vi "Test Power Supply API.vi"() -> ()   [LabVIEW 2025, in "Power Supply.lvlib"]
doc: "Power Supply API Tester.\n\n<b>Note:</b> This VI was modified by the <b>Validate DQMH Module</b> tool to add the 'Show Main VI Diagram on Init' functionality included in DQMH 6.1.\n\n<b>Note:</b> This VI was modified by the <b>Validate DQMH Module</b> tool to upgrade it to the DQMH 5.0 approach to only call the Stop Module.vi at the end of the tester if the module wasn't originally running when the tester started.\n\n<b>Note:</b> This VI was modified by the <b>Validate DQMH Module</b> tool to remove code to stop the main loop on error, and instead display the most recent error on the tester front panel.\n\n<b>Note:</b> This VI was modified by the <b>Validate DQMH Module</b> tool to upgrade its Error Reported event frame to use an improved mechanism for displaying error information."
uses:
  Power Supply.lvlib
  <vilib>/MGI/Panel Manager/Panel/Panel.lvlib
  <vilib>/MGI/Panel Manager/Panel/Panel/Window/Window.vi
  <vilib>/MGI/Panel Manager/Panel/Panel/Window/Window.lvclass
  <vilib>/MGI/Panel Manager/Panel/Panel/Subpanel/Subpanel.vi
  <vilib>/MGI/Panel Manager/Panel/Panel/Subpanel/Subpanel.lvclass
  <vilib>/MGI/Panel Manager/Panel/Panel/Window/Dialog/Dialog.vi
  <vilib>/MGI/Panel Manager/Panel/Panel/Window/Dialog/Dialog.lvclass
  <vilib>/Utility/error.llb/DialogType.ctl
  DC Output--enum.ctl
  Function Generator State--cluster.ctl
  Function Generator Parameters--cluster.ctl
panel:
  in  "Function Generator":T1
  in  "Set Function Generator Parameters":bool
  in  "Function Generator State":T2
  in  "Set Function Generator State":bool
  in  "Disconnect":bool
  in  "Connect":bool
  out "last error":errorcluster
  in  "Show Main VI Diagram on Init (F)":bool
  out "Power Supply State":map{string, dbl}(c390)
  in  "DC Ouput":T3
  in  "Set DC Output":bool
  in  "Plugin File Path":path
  in  "Set Power Supply Plugin":bool
  in  "Power [W]":dbl
  in  "Set Power SP":bool
  in  "Voltage SP [V]":dbl
  in  "Set Voltage SP":bool
  in  "Current SP [A]":dbl
  in  "Set Current SP":bool
  in  "Autoshow?":bool
  in  "Panel Type":enum16{"Window", "Dialog", "Subpanel"}(ring)
  in  "Change Panel":bool
  in  "Tab Control":enum32{"Status", "Subpanel"}(tab)
  out "Status":string
  in  "Show Block Diagram":bool
  in  "Stop Module":bool
  in  "Start Module":bool
  in  "Hide Module Panel":bool
  in  "Show Module Panel":bool
  out "Module Running?":bool
  # "This VI tests the API for the Module."
  # "Change Panel"
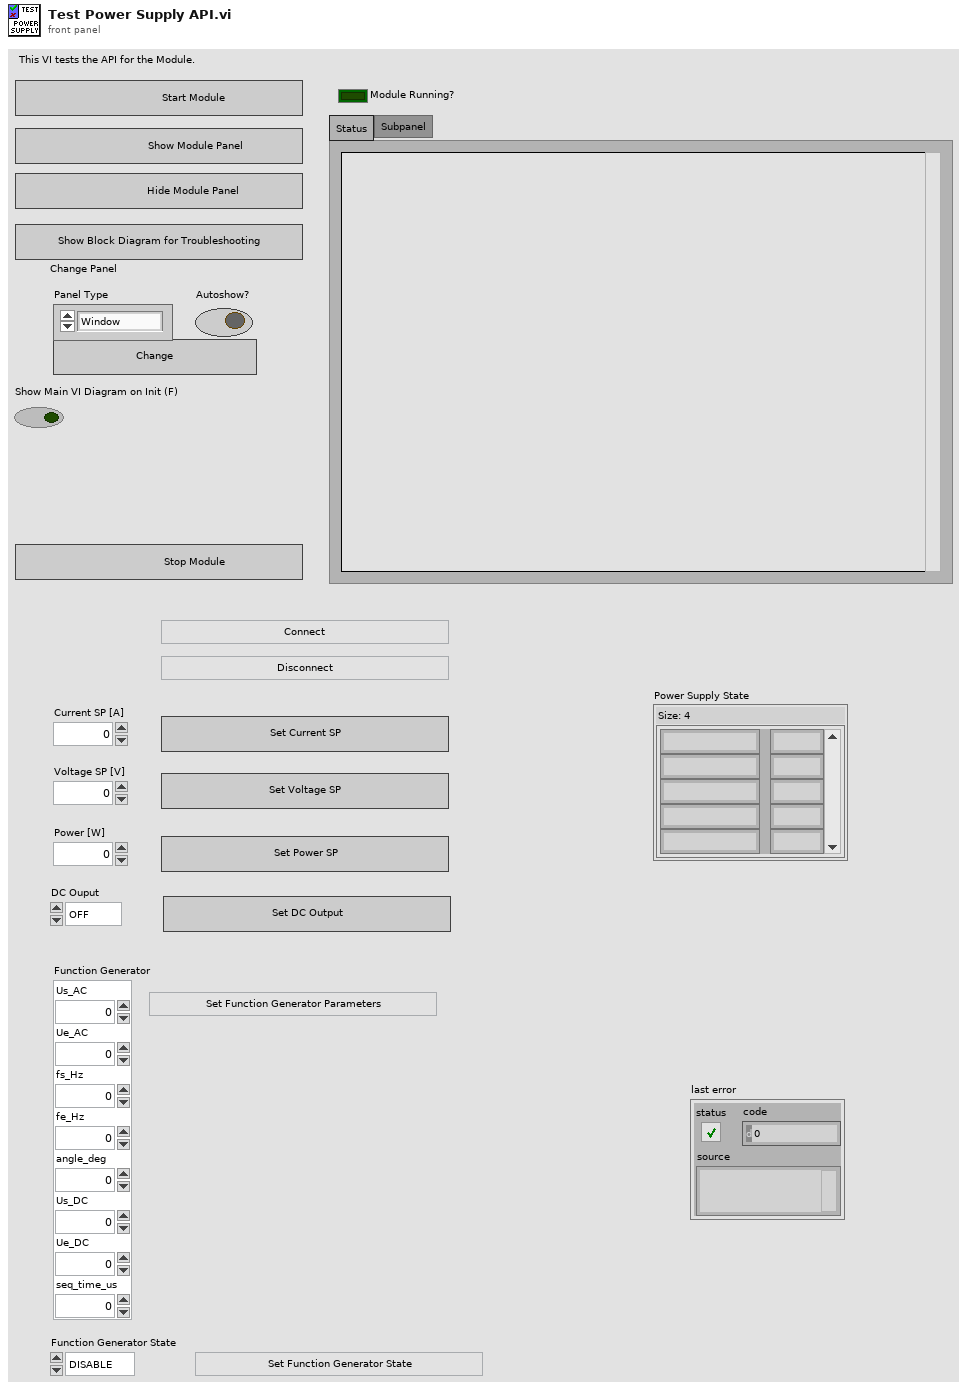
[diagram p1: front panel]
types:
  T1 = typedef "Power Supply.lvlib/Function Generator Parameters--cluster.ctl" = cluster{"Us_AC":sgl, "Ue_AC":sgl, "fs_Hz":sgl, "fe_Hz ":sgl, "angle_deg ":sgl, "Us_DC ":sgl, "Ue_DC":sgl, "seq_time_us":sgl}
  T2 = typedef "Power Supply.lvlib/Function Generator State--cluster.ctl" = enum16{"DISABLE", "ENABLE"}
  T3 = typedef "Power Supply.lvlib/DC Output--enum.ctl" = enum16{"OFF", "ON"}
  T4 = typedef "Power Supply.lvlib/Broadcast Events--cluster.ctl" = cluster{"Module Did Init":refnum<user-event>, "Status Updated":refnum<user-event>, "Error Reported":refnum<user-event>, "Module Did Stop":refnum<user-event>, "Update Module Execution Status":refnum<user-event>, "Broadcast Power Supply State":refnum<user-event>}
  T5 = typedef "DialogType.ctl" = u16
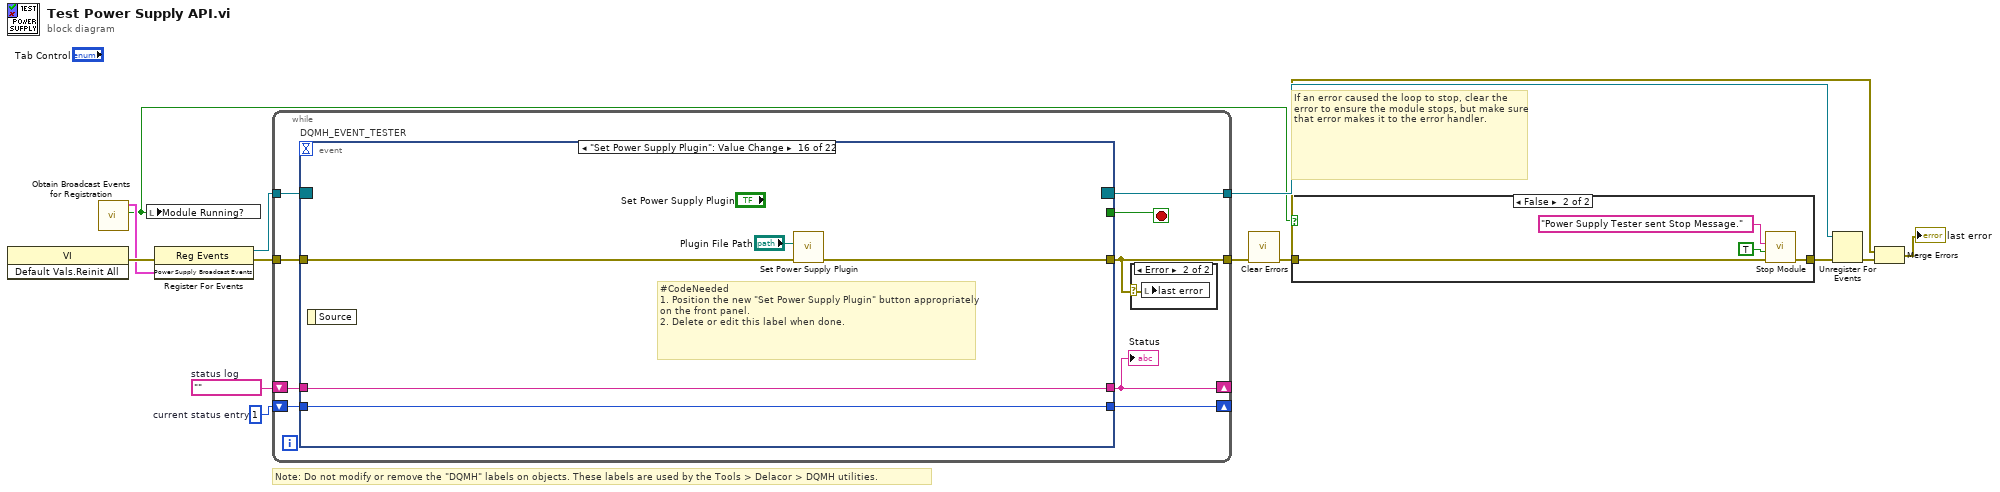
[diagram p0: block diagram]
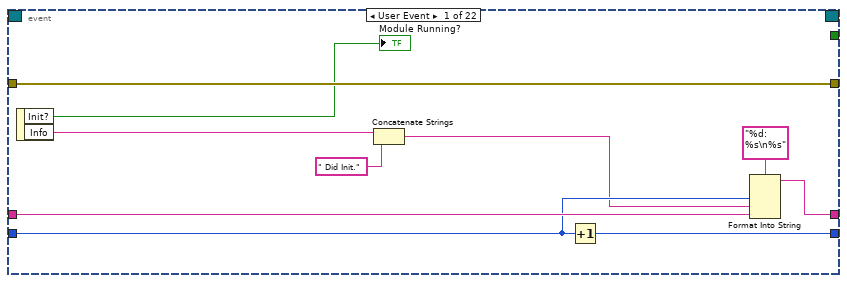
[diagram p4: hidden frame]
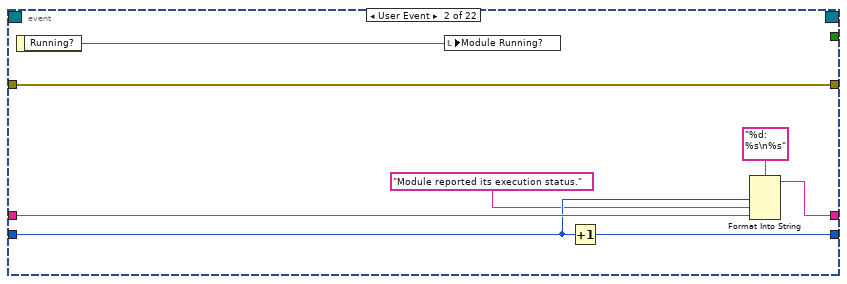
[diagram p5: hidden frame]
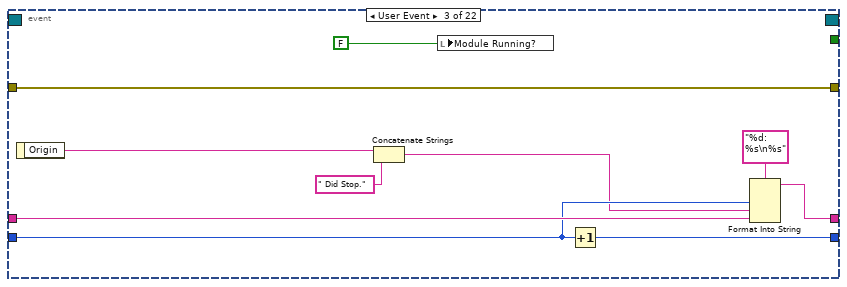
[diagram p6: hidden frame]
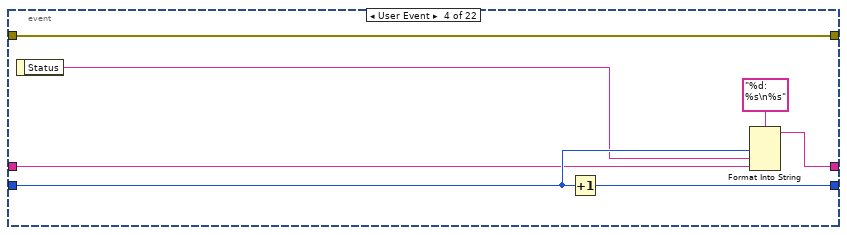
[diagram p7: hidden frame]
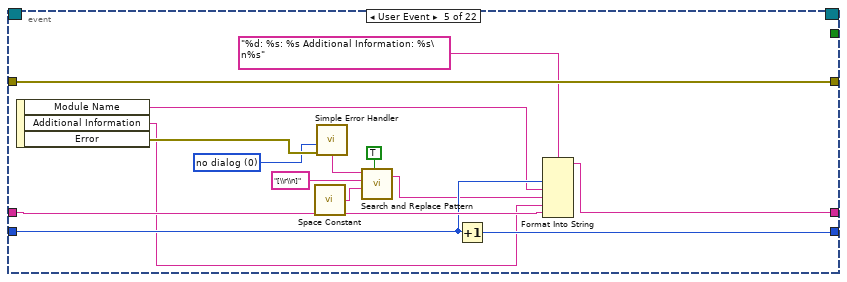
[diagram p8: hidden frame]
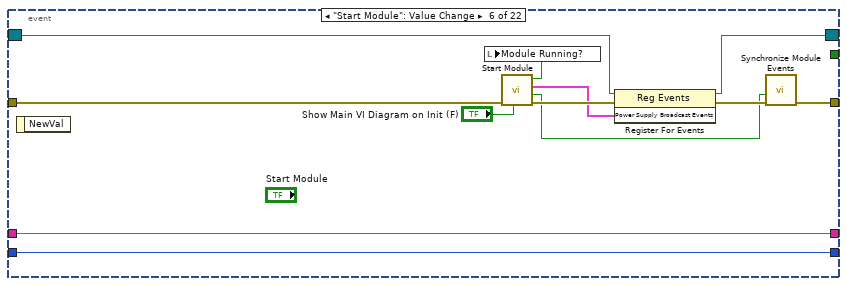
[diagram p9: hidden frame]
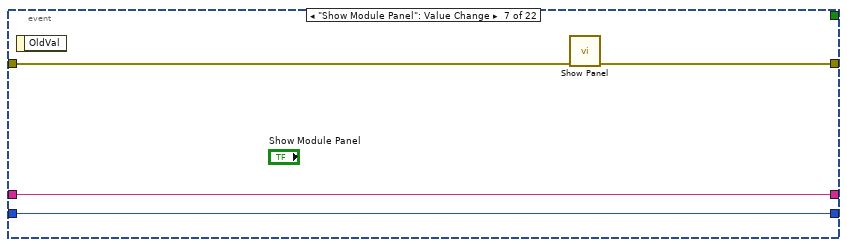
[diagram p10: hidden frame]
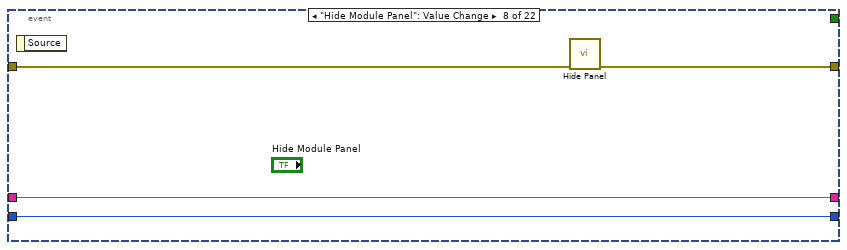
[diagram p11: hidden frame]
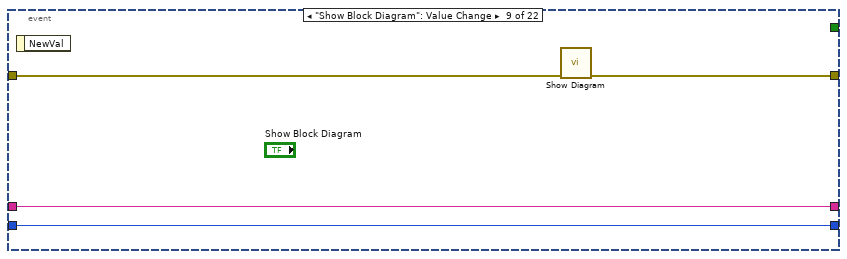
[diagram p12: hidden frame]
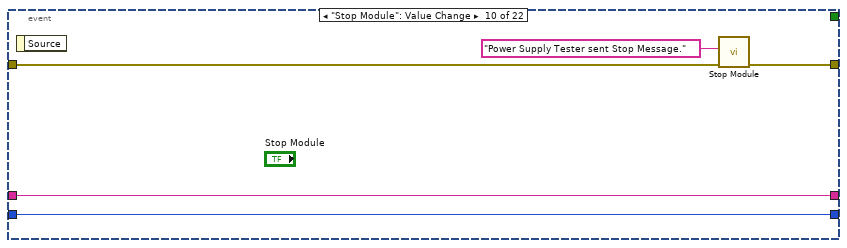
[diagram p13: hidden frame]
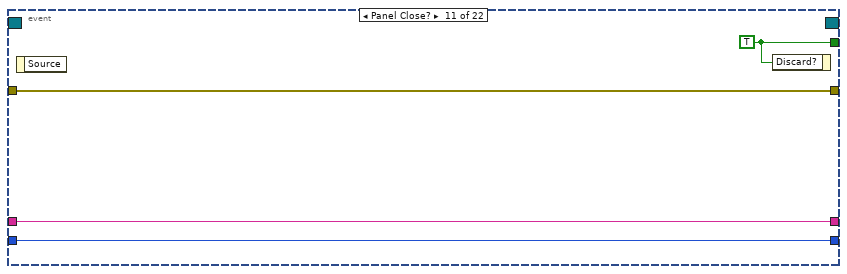
[diagram p14: hidden frame]
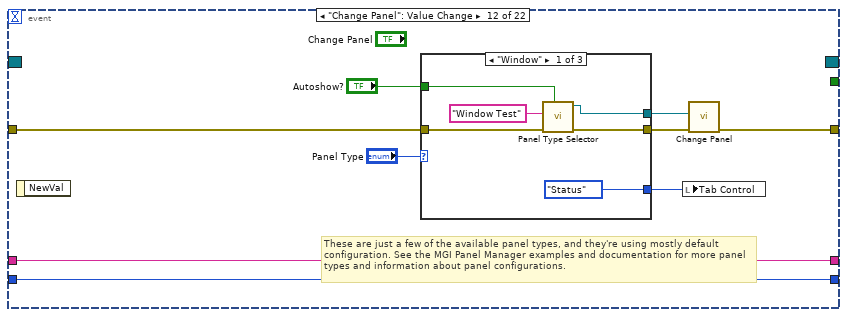
[diagram p15: hidden frame]
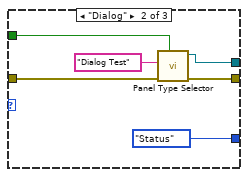
[diagram p16: hidden frame]
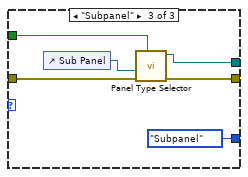
[diagram p17: hidden frame]
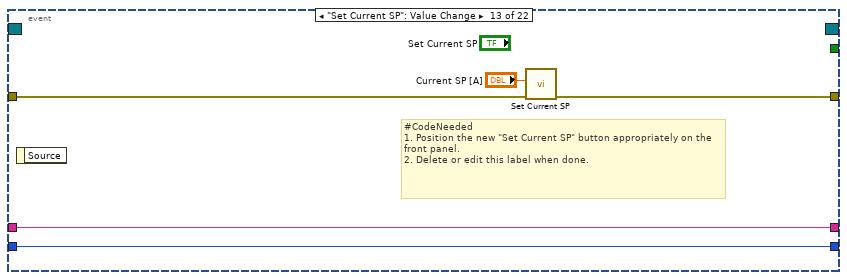
[diagram p18: hidden frame]
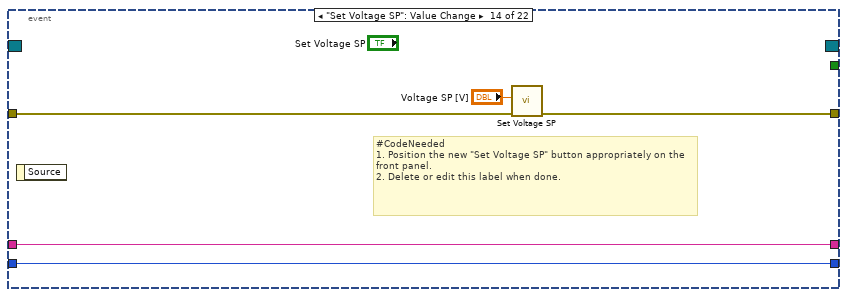
[diagram p19: hidden frame]
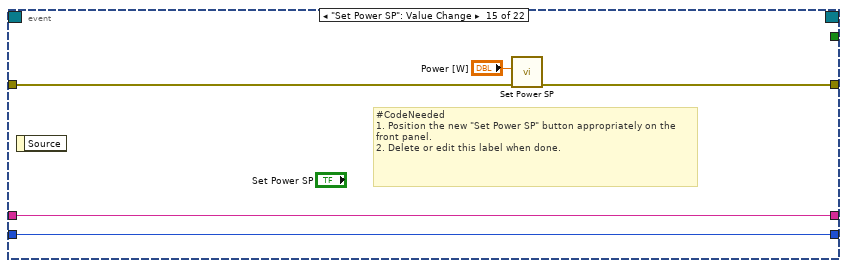
[diagram p20: hidden frame]
diagram:
  w10 = 1  # current status entry
  w11 = ""  # status log
  # "If an error caused the loop to stop, clear the error to ensure the module stops, but make sure that error makes it to the error handler."
  # "Note: Do not modify or remove the \"DQMH\" labels on objects. These labels are used by the Tools > Delacor > DQMH utilities."
  n1 = invoke class="VI" method="Default Vals.Reinit All"() -> (error out=w9:errorcluster)  [unwired: 3 in, 2 out]
  n2 = call "Obtain Broadcast Events for Registration.vi"() -> ("Already running?"=w2:bool, "Power Supply Broadcast Events"=w7:T4)  [unwired: 9 in, 1 out]
  n3 = local write "Module Running?"(w2) -> ()
  n4 = register-events(error in=w9, w7) -> (reference out=w6:refnum<event-registration>, error out=w8:errorcluster)  [unwired: 1 in]
  n5 = while {
    tunnel: w6 -> [w22]
    tunnel: [w15] -> w3
    shift-right: [w18] -> _
    shift-left: w11 -> [w20]
    shift-right: [w19] -> _
    shift-left: w10 -> [w21]
    tunnel: w8 -> [w17]
    tunnel: [w16] -> w5
    stop <- w14 stop-if-true
    n6 = event "DQMH_EVENT_TESTER" shown="[15] \"Set Power Supply Plugin\": Value Change" {
      selector: w22 -> [_ _ _ _ _ w79 _ _ _ _ _ _ _ _ _ _ _ _ _ _ _ _]
      dyn-events: [_ _ _ _ _ w78 _ _ _ _ _ _ _ _ _ _ _ _ _ _ _ _] -> w16
      timeout: _ -> [_ _ _ _ _ _ _ _ _ _ _ _ _ _ _ _ _ _ _ _ _ _]
      tunnel: [_ _ _ _ _ _ _ _ _ _ w106 _ _ _ _ _ _ _ _ _ _ _] -> w14
      tunnel: [w33 w35 w42 w52 w73 w77 w89 w93 w94 w100 w103 w113 w135 w140 w145 w150 w155 w168 w169 w173 w178 w183] -> w15
      tunnel: w21 -> [w29 w39 w49 w55 w70 w82 w87 w91 w95 w101 w104 w114 w136 w141 w146 w151 w156 w165 w170 w174 w179 w184]
      tunnel: w20 -> [w30 w40 w50 w54 w72 w83 w88 w92 w96 w102 w105 w115 w137 w142 w147 w152 w157 w167 w171 w175 w180 w185]
      tunnel: [w27 w37 w47 w56 w71 w83 w88 w92 w96 w102 w105 w115 w137 w142 w147 w152 w157 w166 w171 w175 w180 w185] -> w18
      tunnel: [w28 w38 w48 w58 w69 w82 w87 w91 w95 w101 w104 w114 w136 w141 w146 w151 w156 w164 w170 w174 w179 w184] -> w19
      tunnel: w17 -> [w33 w35 w42 w52 w73 w75 w86 w90 w97 w98 w103 w112 w138 w143 w148 w153 w158 w168 w172 w176 w181 w186]
      event User Event {
        n7 = event-data() -> ("Init?"=→"Module Running?":bool, "Info"=w26:string)  [unwired: 1 in]
        n8 = Concatenate Strings(w26, " Did Init.") -> (w25:string)
        n9 = Increment(x=w29) -> (x+1=w28:i32)
        n10 = Format Into String(format string="%d: %s\n%s", w29, w25, w30) -> (resulting string=w27:string)  [unwired: 2 in, 1 out]
      }
      event User Event {
        n11 = event-data() -> ("Running?"=w34:bool)  [unwired: 1 in]
        n12 = local write "Module Running?"(w34) -> ()
        n13 = Increment(x=w39) -> (x+1=w38:i32)
        n14 = Format Into String(format string="%d: %s\n%s", w39, "Module reported its execution status.", w40) -> (resulting string=w37:string)  [unwired: 2 in, 1 out]
      }
      event User Event {
        n15 = event-data() -> ("Origin"=w46:string)  [unwired: 1 in]
        n16 = Concatenate Strings(w46, " Did Stop.") -> (w45:string)
        n17 = local write "Module Running?"(FALSE ("Module Did Init?")) -> ()
        n18 = Increment(x=w49) -> (x+1=w48:i32)
        n19 = Format Into String(format string="%d: %s\n%s", w49, w45, w50) -> (resulting string=w47:string)  [unwired: 2 in, 1 out]
      }
      event User Event {
        n20 = event-data() -> ("Status"=w53:string)  [unwired: 1 in]
        n21 = Increment(x=w55) -> (x+1=w58:i32)
        n22 = Format Into String(format string="%d: %s\n%s", w55, w53, w54) -> (resulting string=w56:string)  [unwired: 2 in, 1 out]
      }
      event User Event {
        w65 = T5 0 items=["no dialog", "OK message", "continue or stop message", "OK message + warnings", "continue/stop + warnings"] ("type of dialog (OK msg:1)")
        n23 = event-data() -> ("Module Name"=w66:string, "Additional Information"=w67:string, "Error"=w68:errorcluster)  [unwired: 1 in]
        n24 = call <vilib>:"Space Constant.vi"() -> ("String"=w61:string)
        n25 = call <vilib>:"Simple Error Handler.vi"("type of dialog (OK msg:1)"=w65, "error in (no error)"=w68) -> ("message"=w64:string)  [unwired: 3 in, 4 out]
        n26 = call <vilib>:"Search and Replace Pattern.vi"("string"=w64, "regular expression (\"\")"="[\\r\\n]" ("regular expression (\"\")"), "replace string (\"\")"=w61, "replace all? (F)"=TRUE ("replace all CR/LF with spaces")) -> ("result string"=w63:string)  [unwired: 1 in, 1 out]
        n27 = Increment(x=w70) -> (x+1=w69:i32)
        n28 = Format Into String(format string="%d: %s: %s Additional Information: %s\n%s", w70, w66, w63, w67, w72) -> (resulting string=w71:string)  [unwired: 2 in, 1 out]
      }
      event "Start Module": Value Change {
        n29 = event-data() -> ()  [unwired: 1 in, 1 out]
        n30 = call "Start Module.vi"("Show Main VI Diagram on Init (F)"="Show Main VI Diagram on Init (F)", "error in (no error)"=w75) -> ("error out"=w84:errorcluster, "Wait for Event Sync?"=w81:bool, "Power Supply Broadcast Events"=w80:T4, "Module Was Already Running?"=w76:bool)  [unwired: 6 in]
        n31 = local write "Module Running?"(w76) -> ()
        n32 = register-events(reference=w79, error in=w84, w80) -> (reference out=w78:refnum<event-registration>, error out=w85:errorcluster)
        n33 = call "Synchronize Module Events.vi"("error in (no error)"=w85, "Wait for Event Sync?"=w81) -> ("error out"=w77:errorcluster)  [unwired: 9 in]
      }
      event "Show Module Panel": Value Change {
        n34 = event-data() -> ()  [unwired: 1 in, 1 out]
        n35 = call "Show Panel.vi"("error in (no error)"=w86) -> ("error out"=w89:errorcluster)  [unwired: 10 in]
      }
      event "Hide Module Panel": Value Change {
        n36 = event-data() -> ()  [unwired: 1 in, 1 out]
        n37 = call "Hide Panel.vi"("error in (no error)"=w90) -> ("error out"=w93:errorcluster)  [unwired: 10 in]
      }
      event "Show Block Diagram": Value Change {
        n38 = event-data() -> ()  [unwired: 1 in, 1 out]
        n39 = call "Show Diagram.vi"("error in (no error)"=w97) -> ("error out"=w94:errorcluster)  [unwired: 10 in]
      }
      event "Stop Module": Value Change {
        n40 = event-data() -> ()  [unwired: 1 in, 1 out]
        n41 = call "Stop Module.vi"("error in (no error)"=w98, "Origin"="Power Supply Tester sent Stop Message.") -> ("error out"=w100:errorcluster)  [unwired: 9 in]
      }
      event Panel Close? {
        w106 = TRUE ("Discard?")
        n42 = event-data() -> ()  [unwired: 1 in, 1 out]
        n43 = event-data("Discard?"=w106) -> ()  [unwired: 1 in, 1 out]
      }
      event "Change Panel": Value Change {
        # "These are just a few of the available panel types, and they're using mostly default configuration. See the MGI Panel Manager examples and documentation for more panel types and information about panel configurations."
        n44 = event-data() -> ()  [unwired: 1 in, 1 out]
        n45 = case shown="\"Window\"" "Panel Type" {
          tunnel: w112 -> [w121 w127 w133]
          tunnel: [w120 w126 w132] -> w111
          tunnel: [w119 w125 w131] -> w110
          tunnel: [enum32{"Status", "Subpanel"}."Status" ("Tab Control") enum32{"Status", "Subpanel"}."Status" ("Tab Control") enum32{"Status", "Subpanel"}."Subpanel" ("Tab Control")] -> w108
          tunnel: "Autoshow?" -> [w116 w122 w128]
          frame "Window" {
            n46 = call-poly <vilib>:"Panel Type Selector.vi"("Autoshow? (T)"=w116, "error in (no error)"=w121, "Default Title"="Window Test") -> ("error out"=w120:errorcluster, "Window out"=w119:refnum<class "Window.lvclass">)  [unwired: 7 in]
          }
          frame "Dialog" {
            n47 = call-poly <vilib>:"Panel Type Selector.vi"("Autoshow? (T)"=w122, "Error In"=w127, "Default Title"="Dialog Test") -> ("Error Out"=w126:errorcluster, "Dialog out"=w125:refnum<class "Dialog.lvclass">)  [unwired: 7 in]
          }
          frame "Subpanel" {
            n48 = control-ref of="Sub Panel"() -> (w130:refnum<vi>)
            n49 = call-poly <vilib>:"Panel Type Selector.vi"("Autoshow? (T)"=w128, "Error In"=w133, "Sub Panel"=w130) -> ("Error Out"=w132:errorcluster, "Subpanel Out"=w131:refnum<class "Subpanel.lvclass">)  [unwired: 7 in]
          }
        }
        n50 = local write "Tab Control"(w108) -> ()
        n51 = call "Change Panel.vi"("error in (no error)"=w111, "New Panel"=w110) -> ("error out"=w113:errorcluster)  [unwired: 9 in]
      }
      event "Set Current SP": Value Change {
        # "#CodeNeeded\n1. Position the new \"Set Current SP\" button appropriately on the front panel.\n2. Delete or edit this label when done."
        n52 = event-data() -> ()  [unwired: 1 in, 1 out]
        n53 = call "Set Current SP.vi"("error in"=w138, "Current SP [A]"="Current SP [A]") -> ("error out"=w135:errorcluster)  [unwired: 9 in]
      }
      event "Set Voltage SP": Value Change {
        # "#CodeNeeded\n1. Position the new \"Set Voltage SP\" button appropriately on the front panel.\n2. Delete or edit this label when done."
        n54 = event-data() -> ()  [unwired: 1 in, 1 out]
        n55 = call "Set Voltage SP.vi"("error in"=w143, "Voltage SP [V]"="Voltage SP [V]") -> ("error out"=w140:errorcluster)  [unwired: 9 in]
      }
      event "Set Power SP": Value Change {
        # "#CodeNeeded\n1. Position the new \"Set Power SP\" button appropriately on the front panel.\n2. Delete or edit this label when done."
        n56 = event-data() -> ()  [unwired: 1 in, 1 out]
        n57 = call "Set Power SP.vi"("error in"=w148, "Power [W]"="Power [W]") -> ("error out"=w145:errorcluster)  [unwired: 9 in]
      }
      event "Set Power Supply Plugin": Value Change {
        # "#CodeNeeded\n1. Position the new \"Set Power Supply Plugin\" button appropriately on the front panel.\n2. Delete or edit this label when done."
        n58 = event-data() -> ()  [unwired: 1 in, 1 out]
        n59 = call "Set Power Supply Plugin.vi"("error in"=w153, "Plugin File Path"="Plugin File Path") -> ("error out"=w150:errorcluster)  [unwired: 9 in]
      }
      event "Set DC Output": Value Change {
        n60 = event-data() -> ()  [unwired: 1 in, 1 out]
        n61 = call "Set DC Output.vi"("error in"=w158, "DC Ouput"="DC Ouput") -> ("error out"=w155:errorcluster)  [unwired: 9 in]
      }
      event User Event {
        # "#CodeNeeded Replace this format string with a meaningful value for this broadcast, then wire broadcast data from the Event Data Node to the input(s) of the Format Into String function."
        # "#CodeNeeded\n1. Process the event data sent by the \"Broadcast Power Supply State\" broadcast event.\n2. Delete or edit this label when done."
        n62 = event-data() -> ("Power Supply State"=→"Power Supply State":map{string, dbl})  [unwired: 1 in, 4 out]
        n63 = Format Into String(format string="Response Received - %s", "Power supply state map recieved." ("input 1")) -> (resulting string=w161:string)  [unwired: 2 in, 1 out]
        n64 = Increment(x=w165) -> (x+1=w164:i32)
        n65 = Format Into String(format string="%d: %s\n%s", w165, w161, w167) -> (resulting string=w166:string)  [unwired: 2 in, 1 out]
      }
      event "Connect": Value Change {
        # "#DQMH_CodeNeeded\n1. Position the new \"Connect\" button appropriately on the front panel.\n2. Delete or edit this label when done."
        n66 = event-data() -> ()  [unwired: 1 in, 1 out]
        n67 = call "Connect.vi"("error in"=w172) -> ("error out"=w169:errorcluster)  [unwired: 10 in]
      }
      event "Disconnect": Value Change {
        # "#DQMH_CodeNeeded\n1. Position the new \"Disconnect\" button appropriately on the front panel.\n2. Delete or edit this label when done."
        n68 = event-data() -> ()  [unwired: 1 in, 1 out]
        n69 = call "Disconnect.vi"("error in"=w176) -> ("error out"=w173:errorcluster)  [unwired: 10 in]
      }
      event "Set Function Generator State": Value Change {
        # "#DQMH_CodeNeeded\n1. Position the new \"Set Function Generator State\" button appropriately on the front panel.\n2. Delete or edit this label when done."
        n70 = event-data() -> ()  [unwired: 1 in, 1 out]
        n71 = call "Set Function Generator State.vi"("error in"=w181, "Function Generator State"="Function Generator State") -> ("error out"=w178:errorcluster)  [unwired: 9 in]
      }
      event "Set Function Generator Parameters": Value Change {
        n72 = event-data() -> ()  [unwired: 1 in, 1 out]
        n73 = call "Set Function Generator Parameters.vi"("error in"=w186, "Function Generator"="Function Generator") -> ("error out"=w183:errorcluster)  [unwired: 9 in]
      }
    }
    "Status" <- w18
    n74 = case "DQMH_TESTER_ERROR_LOCAL" shown="Error" w15 {
      selector: w15 -> [_ w23]
      frame No Error {
      }
      frame Error {
        n75 = local write "last error"(w23) -> ()
      }
    }
  }
  n76 = call <vilib>:"Clear Errors.vi"("error in (no error)"=w3) -> ("error out"=w4:errorcluster)  [unwired: 5 in, 1 out]
  n77 = case shown="False" w2 {
    tunnel: [w187 w191] -> w12
    tunnel: w4 -> [w187 w188]
    frame True {
    }
    frame False {
      n78 = call "Stop Module.vi"("error in (no error)"=w188, "Wait for Module to Stop? (F)"=TRUE ("Wait for Module to stop?"), "Origin"="Power Supply Tester sent Stop Message.") -> ("error out"=w191:errorcluster)  [unwired: 8 in]
    }
  }
  n79 = Unregister For Events(event registration refnum=w5, error in=w12) -> (error out=w13:errorcluster)
  n80 = Merge Errors(w3, w13) -> (→"last error":errorcluster)
